vi "StressDist_table.vi"(7 "StressDist_types":T7, 8 "Error In":errorcluster, 11 "main_FGV_data":T1={"pipe_properties"={"out_radius"=0.0, "in_radius"=0.0, "out_diameter"=0.0, "in_diameter"=0.0, "thickness"=0.0, "inertia"=0.0, "area"=0.0}, "DirPath"=path "L:/Documentos/00 SERVIÇOS/Tensão residual/Olapa 10-2017/Dados/Primeira Seção/Furos", "DirReport"=path "L:/Documentos/00 SERVIÇOS/Tensão residual/Olapa 10-2017/RelatóriosOlapa/Teste", "Points"=[], "ovalization_data"={"AngOval"=[0.0, 60.0, 120.0, 22.5, 45.0, 67.5, 90.0, 112.5, 135.0, 157.5, 180.0], "OvalDiam"=[324.25, 324.6, 324.55, 324.25, 324.55, 324.65, 324.6, 324.65, 324.55, 324.5, 324.4], "Plots"={"Ref"={"X"=[], "Y"=[]}, "Elipse"={"X"=[], "Y"=[]}, "Points"={"X"=[], "Y"=[]}}, "Ampliation"=100.0, "Results"={"MD"=0.0, "mD"=0.0, "Dmed"=0.0, "Oval"=0.0, "ang"=0.0, "X0"=0.0, "Y0"=0.0}}, "StressDist_data"={"Long"={"Plot"=[], "Fit"=[], "ColorMap"=[], "Data"=[]}, "Circ"={"Plot"=[], "Fit"=[], "ColorMap"=[], "Data"=[]}, "Shear"={"Plot"=[], "Fit"=[], "ColorMap"=[], "Data"=[]}}}) -> (0 "Error Out":errorcluster, 3 "main_FGV_data-out":T1={"pipe_properties"={"out_radius"=0.0, "in_radius"=0.0, "out_diameter"=0.0, "in_diameter"=0.0, "thickness"=0.0, "inertia"=0.0, "area"=0.0}, "DirPath"=path "L:/Documentos/00 SERVIÇOS/Tensão residual/Olapa 10-2017/Dados/Primeira Seção/Furos", "DirReport"=path "L:/Documentos/00 SERVIÇOS/Tensão residual/Olapa 10-2017/RelatóriosOlapa/Teste", "Points"=[], "ovalization_data"={"AngOval"=[0.0, 60.0, 120.0, 22.5, 45.0, 67.5, 90.0, 112.5, 135.0, 157.5, 180.0], "OvalDiam"=[324.25, 324.6, 324.55, 324.25, 324.55, 324.65, 324.6, 324.65, 324.55, 324.5, 324.4], "Plots"={"Ref"={"X"=[], "Y"=[]}, "Elipse"={"X"=[], "Y"=[]}, "Points"={"X"=[], "Y"=[]}}, "Ampliation"=100.0, "Results"={"MD"=0.0, "mD"=0.0, "Dmed"=0.0, "Oval"=0.0, "ang"=0.0, "X0"=0.0, "Y0"=0.0}}, "StressDist_data"={"Long"={"Plot"=[], "Fit"=[], "ColorMap"=[], "Data"=[]}, "Circ"={"Plot"=[], "Fit"=[], "ColorMap"=[], "Data"=[]}, "Shear"={"Plot"=[], "Fit"=[], "ColorMap"=[], "Data"=[]}}})   [LabVIEW 2016]
uses:
  StressDist_types.ctl
  MainFGV/main_FGV_data.ctl
  MainFGV/pipe_properties.ctl
  StressCalculations/point_data.ctl
  Ovalization/ovalization_data.ctl
  StressDist_data.ctl
  StressDist_single_data.ctl
  Report/report_mods.ctl
  <vilib>/Analysis/baseanly.llb/Mean (DBL).vi
  <vilib>/Analysis/NI_AALBase.lvlib
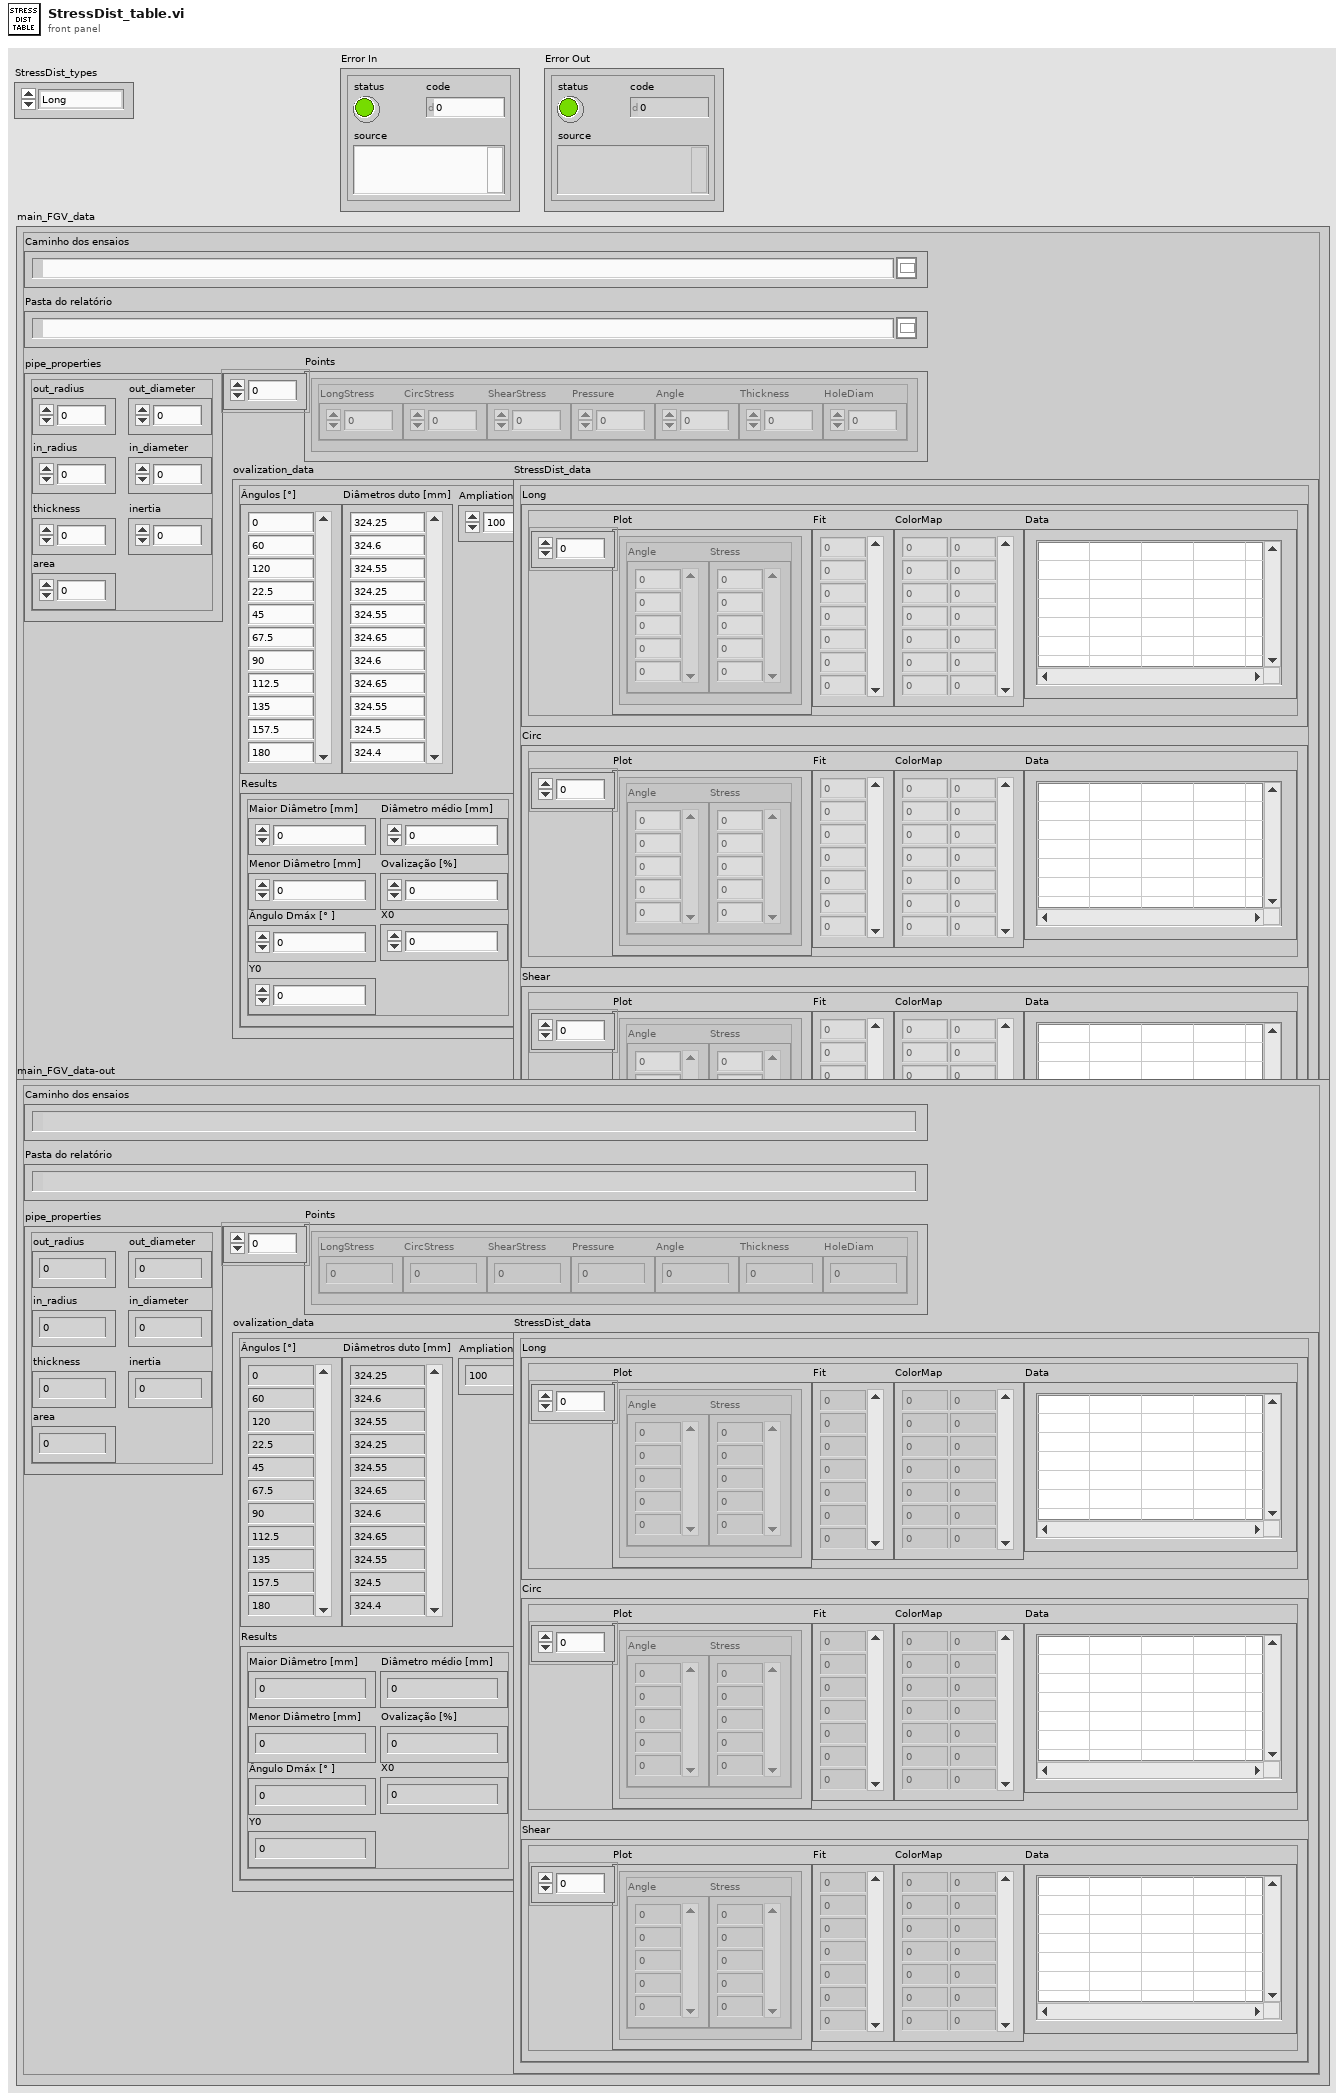
[diagram p1: front panel]
types:
  T1 = typedef "main_FGV_data.ctl" = cluster{"pipe_properties":T2, "DirPath":path, "DirReport":path, "Points":T3[], "ovalization_data":T4, "StressDist_data":T5}
  T2 = typedef "pipe_properties.ctl" = cluster{"out_radius":dbl, "in_radius":dbl, "out_diameter":dbl, "in_diameter":dbl, "thickness":dbl, "inertia":dbl, "area":dbl}
  T3 = typedef "point_data.ctl" = cluster{"LongStress":dbl, "CircStress":dbl, "ShearStress":dbl, "Pressure":dbl, "Angle":dbl, "Thickness":dbl, "HoleDiam":dbl}
  T4 = typedef "ovalization_data.ctl" = cluster{"AngOval":dbl[], "OvalDiam":dbl[], "Plots":cluster{"Ref":cluster{"X":dbl[], "Y":dbl[]}, "Elipse":cluster{"X":dbl[], "Y":dbl[]}, "Points":cluster{"X":dbl[], "Y":dbl[]}}, "Ampliation":dbl, "Results":cluster{"MD":dbl, "mD":dbl, "Dmed":dbl, "Oval":dbl, "ang":dbl, "X0":dbl, "Y0":dbl}}
  T5 = typedef "StressDist_data.ctl" = cluster{"Long":T6, "Circ":T6, "Shear":T6}
  T6 = typedef "StressDist_single_data.ctl" = cluster{"Plot":cluster{"Angle":dbl[], "Stress":dbl[]}[], "Fit":dbl[], "ColorMap":dbl[][], "Data":string[][]}
  T7 = typedef "StressDist_types.ctl" = enum16{"Long", "Circ", "Shear"}
  T8 = typedef "report_mods.ctl" = enum16{"Init", "Table", "Graph", "End"}
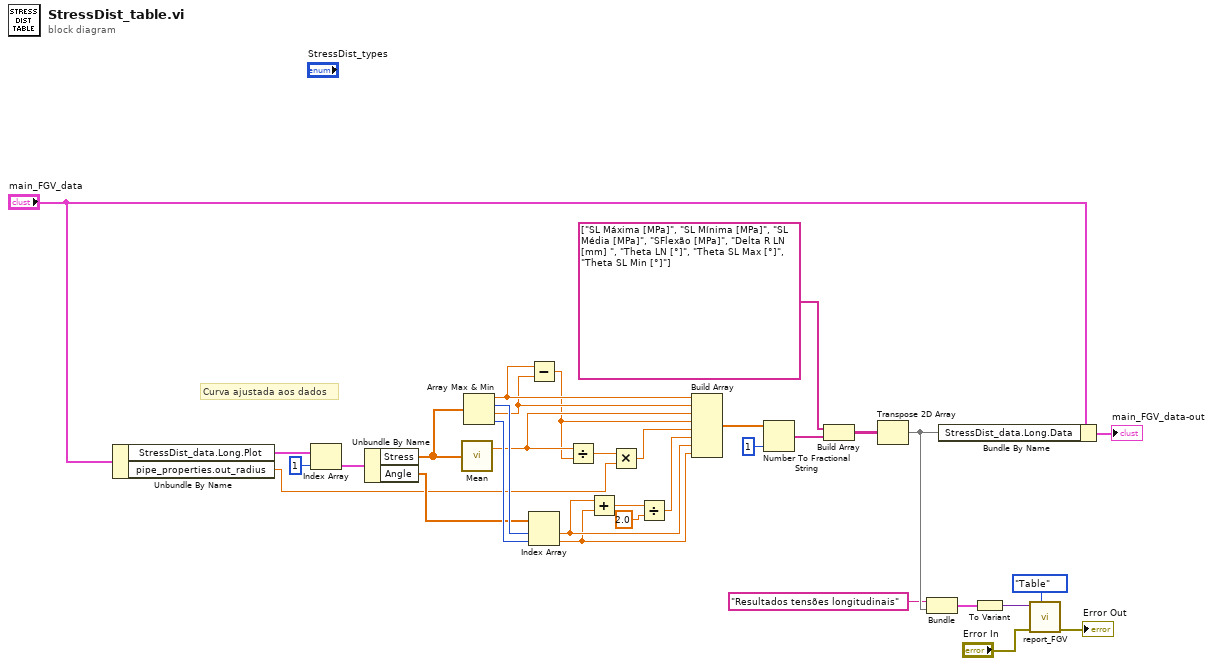
[diagram p0: block diagram]
diagram:
  # "Curva ajustada aos dados"
  n1 = Unbundle By Name("main_FGV_data") -> ("StressDist_data.Long.Plot"=w33:cluster{"Angle":dbl[], "Stress":dbl[]}[], "pipe_properties.out_radius"=w16:dbl)
  n2 = Index Array(array=w33, index=1) -> (element=w31:cluster{"Angle":dbl[], "Stress":dbl[]})
  n3 = Unbundle By Name(w31) -> ("Stress"=w30:dbl[], "Angle"=w27:dbl[])
  n4 = call-poly <vilib>:"Mean.vi"("X"=w30) -> ("mean"=w19:dbl)  [unwired: 1 out]
  n5 = Array Max & Min(array=w30) -> (max value=w21:dbl, max index (indices)=w29:i32, min value=w20:dbl, min index (indices)=w28:i32)
  n6 = Subtract(x=w21, y=w20) -> (x-y=w18:dbl)
  n7 = Index Array(array=w27, index #1=w29, index #2=w28) -> (element #1=w26:dbl, element #2=w25:dbl)
  n8 = Divide(x=w19, y=w18) -> (x/y=w17:dbl)
  n9 = Add(x=w26, y=w25) -> (x+y=w24:dbl)
  n10 = Multiply(x=w17, y=w16) -> (x*y=w15:dbl)
  n11 = Divide(x=w24, y=2.0) -> (x/y=w22:dbl)
  n12 = Build Array(w21, w20, w19, w18, w15, w22, w26, w25) -> (w14:dbl[])
  n13 = Number To Fractional String(number=w14, precision (6)=i16 1) -> (F-format string=w12:string[])  [unwired: 2 in]
  n14 = Build Array(string[] ["SL Máxima [MPa]", "SL Mínima [MPa]", "SL Média [MPa]", "SFlexão [MPa]", "Delta R LN [mm] ", "Theta LN [°]", "Theta SL Max [°]", "Theta SL Min [°]"], w12) -> (w10:string[][])
  n15 = Transpose 2D Array(2D array=w10) -> (transposed array=w6:string[][])
  n16 = Bundle("Resultados tensões longitudinais", w6) -> (w4:cluster{string, string[][]})  [unwired: 1 in]
  n17 = Bundle By Name(cluster="main_FGV_data", "StressDist_data.Long.Data"=w6) -> (→"main_FGV_data-out":T1)
  n18 = To Variant(anything=w4) -> (Variant=w3:variant)
  n19 = call "report_FGV.vi"("report_mods"=report_mods."Table", "Error In"="Error In", "Data in"=w3) -> ("Error Out"=→"Error Out":errorcluster)  [unwired: 8 in]
